vi "get-video-ROIs.vi"() -> ()   [LabVIEW 2024]
uses:
  <vilib>/vision/NI_Vision_Development_Module.lvlib
panel:
  out "ROI Descriptor out":T1 {"Contours"."Type" items=["No Selection", "Point", "Line", "Rectangle", "Oval", "Polygon", "Freehand Region", "Annulus", "Unused2", "Unused3", "Broken Line", "Freehand Line", "Rotated Rectangle"]}
  out "ROI Descriptors out":T1[](array[typedef]) {"Contours"."Type" items=["No Selection", "Point", "Line", "Rectangle", "Oval", "Polygon", "Freehand Region", "Annulus", "Unused2", "Unused3", "Broken Line", "Freehand Line", "Rotated Rectangle"]}
  in  "stop":bool
  out "Gray Image":T2(plugin-control)
  out "Image Out":T2(plugin-control)
  out "error out":errorcluster
  out "ROI manual":T2(plugin-control)
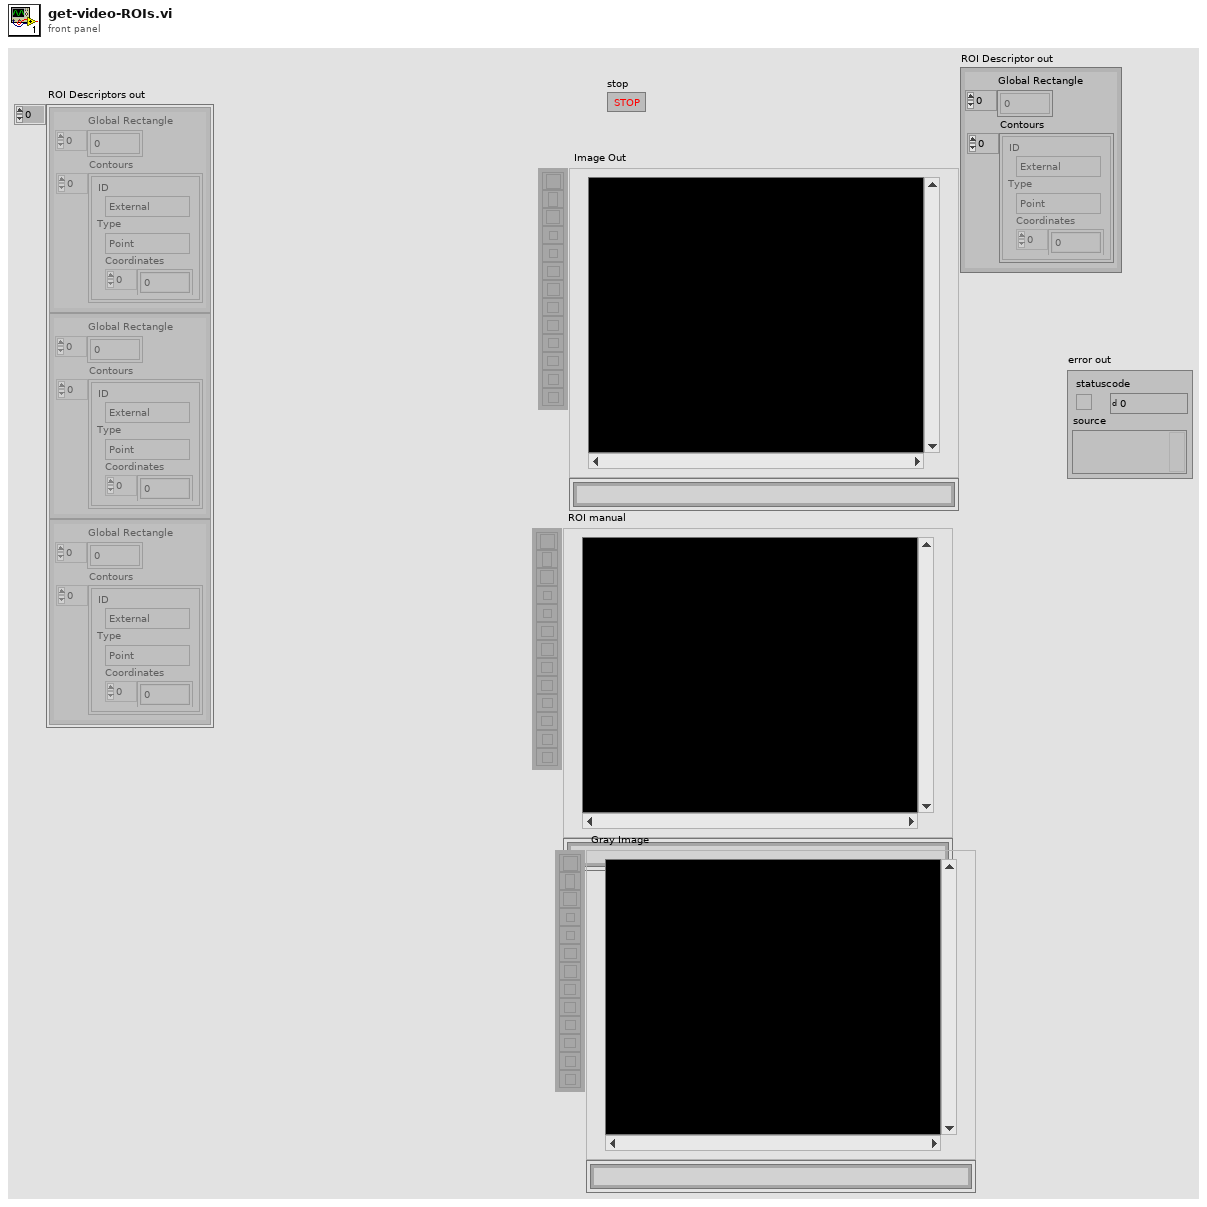
[diagram p1: front panel]
types:
  T1 = typedef "ROI Descriptor" = cluster{"Global Rectangle":i32[], "Contours":cluster{"ID":enum32{"External", "Internal"}, "Type":u32, "Coordinates":i32[]}[]}
  T2 = typedef "IMAQ Image.ctl" = refnum<image>
  T3 = typedef "Image Type" = u32
  T4 = cluster{"Global Rectangle":i32[], "Contours":cluster{"Contour Type":u32, "ROI Type":u32, "Points":i32[]}[]}
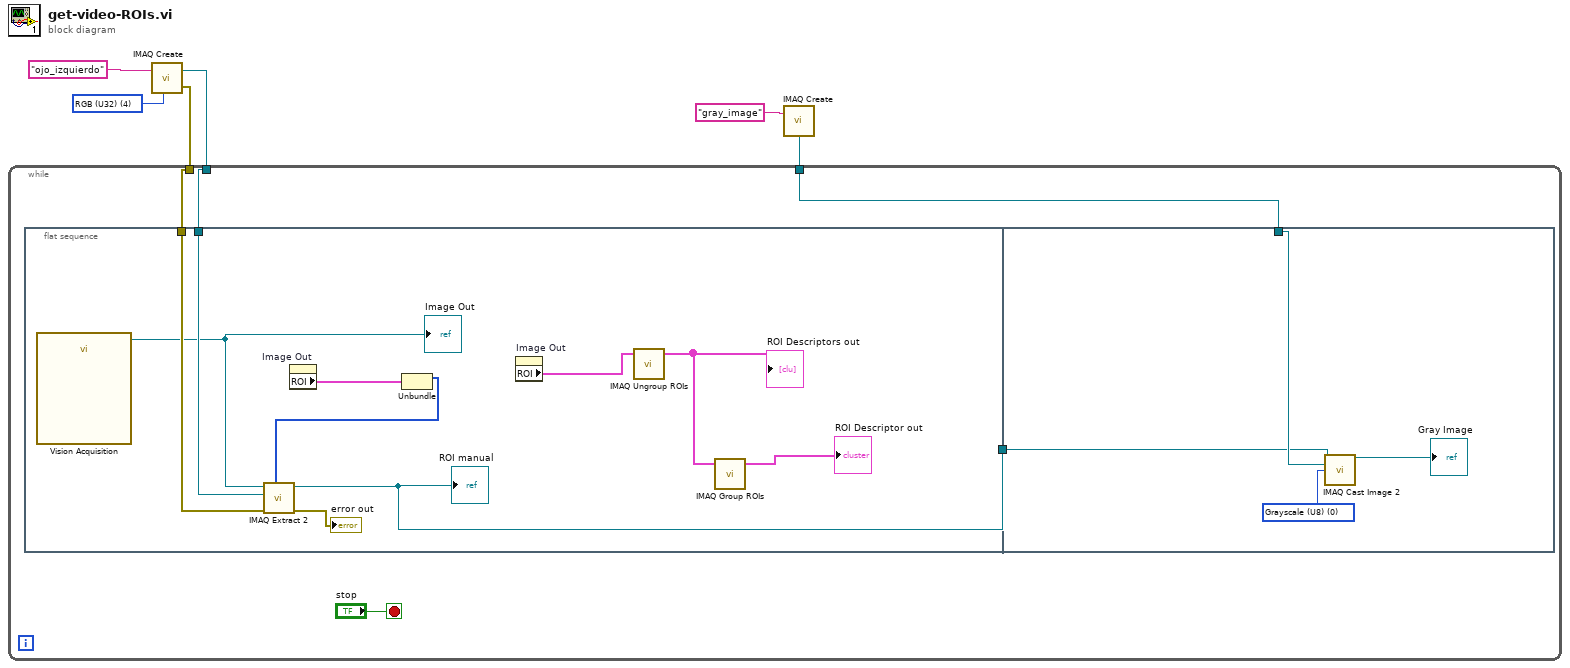
[diagram p0: block diagram]
diagram:
  w5 = T3 4 items=["Grayscale (U8)", "Grayscale (I16)", "Grayscale (SGL)", "Complex (CSG)", "RGB (U32)", "HSL (U32)", "RGB (U64)", "Grayscale (U16)"] ("Image Type")
  n1 = call "IMAQ Create"("Image Name"="ojo_izquierdo", "Image Type"=w5) -> ("New Image"=w3:T2, "error out"=w4:errorcluster)  [unwired: 3 in]
  n2 = call "IMAQ Create"("Image Name"="gray_image") -> ("New Image"=w1:T2)  [unwired: 4 in, 1 out]
  n3 = while {
    tunnel: w4 -> [w10]
    tunnel: w3 -> [w9]
    tunnel: w1 -> [w8]
    stop <- "stop" stop-if-true
    n4 = flat-sequence {
      tunnel: w10 -> [w18]
      tunnel: w9 -> [w17]
      tunnel: [w15] -> w7
      tunnel: w8 -> [w25]
      tunnel: w7 -> [w24]
      frame #0 {
        n5 = call "Vision Acquisition"() -> ("Image Out"=w16:T2)  [unwired: 25 in, 2 out]
        "Image Out" <- w16
        n6 = property on="Image Out" class="ImageControl"() -> ("ROI"=w21:T4)  [unwired: 2 in, 2 out]
        n7 = Unbundle "Unbundle"(w21) -> ("Global Rectangle"=w20:i32[])  [unwired: 1 out]
        n8 = call "IMAQ Extract 2"("Optional Rectangle"=w20, "error in (no error)"=w18, "Image Dst"=w17, "Image Src"=w16) -> ("error out"=→"error out":errorcluster, "Image Dst Out"=w15:T2)  [unwired: 6 in]
        "ROI manual" <- w15
        n9 = property on="Image Out" class="ImageControl"() -> ("ROI"=w14:T4)  [unwired: 2 in, 2 out]
        n10 = call "IMAQ Ungroup ROIs"("ROI Descriptor"=w14) -> ("ROI Descriptors out"=w13:T1[])  [unwired: 3 in, 1 out]
        "ROI Descriptors out" <- w13
        n11 = call "IMAQ Group ROIs"("ROI Descriptors"=w13) -> ("ROI Descriptor out"=→"ROI Descriptor out":T1)  [unwired: 3 in, 1 out]
      }
      frame #1 {
        w23 = T3 0 items=["Grayscale (U8)", "Grayscale (I16)", "Grayscale (SGL)", "Complex (CSG)", "RGB (U32)", "HSL (U32)", "RGB (U64)", "Grayscale (U16)"] ("Image Type")
        n12 = call "IMAQ Cast Image 2"("Image Src"=w24, "Image Dst"=w25, "Image Type"=w23) -> ("Image Dst Out"=→"Gray Image":T2)  [unwired: 11 in, 1 out]
      }
    }
  }
